vi "Keithley_pulse.vi"() -> ()   [LabVIEW 2023]
uses:
  <instrlib>/Keithley 24XX/Public/Data/Read (Multiple Points).vi
  <vilib>/Utility/file.llb/Write Delimited Spreadsheet (DBL).vi
  <instrlib>/Keithley 24XX/Keithley 24XX.lvlib
  <vilib>/Analysis/NI_AALBase.lvlib
panel:
  in  "valley milliseconds":u32=10
  in  "path1 (folder + filename)":string="C:\\Users\\Carter Fox\\Documents\\probe data\\haolin\\"
  in  "Clear Plot":bool
  out "V-R":cluster{dbl[], dbl[]}(graph)={[0.0, -0.5, -1.0, -1.5, -2.0, -2.5, -3.0, -3.5, -4.0, -3.5, -3.0, -2.5, -2.0, -1.5, -1.0, -0.5, 0.0, 0.5, 1.0, 1.5, 2.0, 2.5, 3.0, 3.5, 4.0, 3.5, 3.0, 2.5, 2.0, 1.5, 1.0, 0.5, 0.0, 0.0, -0.5, -1.0, -1.5, -2.0, -2.5, -3.0, -3.5, -4.0, -3.5, -3.0, -2.5, -2.0, -1.5, -1.0, -0.5, 0.0, 0.5, 1.0, 1.5, 2.0, 2.5, 3.0, 3.5, 4.0, 3.5, 3.0, 2.5, 2.0, 1.5, 1.0, 0.5, 0.0], [0.19700693041086198, 0.35372319519519807, 0.20753341913223267, 0.3582892343401909, 0.540878164768219, 0.43121315687894823, 0.1754639378748834, 0.002317465841770172, 0.0942357487976551, 0.08408013060688972, -0.1210348054766655, 0.06776629239320756, 0.04069728031754494, -0.04053474152460694, -0.23445252031087876, -0.3108171131461859, -25.74827651977539, -25.785472869873047, -25.82678337097168, -25.68000602722168, -25.46846694946289, -25.3049674987793, -25.380819702148436, -25.68810615539551, -25.51903533935547, -25.389516067504882, -25.12458267211914, -25.099736404418945, -25.550616455078124, -25.390170669555665, -25.549488830566407, -25.412010192871094, 0.08227393236011267, -0.25657982677221297, -0.08616339890286326, -0.01899189129471779, -0.26742409020662306, -0.07599621266126633, -0.11147867683321237, -0.09915755027905107, -0.13367668855935336, 0.060095877200365064, -0.09875441491603851, 0.18304548561573028, 0.24648103043437003, 0.05984655544161797, -0.01924160271883011, -0.14573073834180833, -0.221831959951669, -25.54925956726074, -25.60353775024414, -24.910662841796874, -25.843761825561522, -25.492467880249023, -26.035901641845705, -25.818101501464845, -25.60927963256836, -25.978542709350585, -25.790420913696288, -25.73311767578125, -26.193365859985352, -25.49853630065918, -25.56501159667969, -25.275862884521484, -25.529310989379884, -25.196596527099608]}
  in  "Sample Count":i32=5
  out "R error":dbl=0.15830408316018257 format="%0.2f"
  out "R":dbl=0.19700693041086198 format="%0.2f"
  in  "Source Mode  (0: Voltage)":u16(ring) items=["Voltage", "Current"]
  in  "Compliance  Level":dbl=1e-06
  in  "hill milliseconds":u32=10
  in  "Serial Configuration":T1={"Baud Rate"=9600, "Parity"=0, "Data Bits"=8, "Stop Bits"=10, "Flow Control"=0} {"Flow Control" items=["None", "XON/XOFF", "RTS/CTS", "XON/XOFF & RTS/CTS", "DTR/DSR", "XON/XOFF & DTR/DSR"]; "Stop Bits" items=["1.0"=10, "1.5"=15, "2.0"=20]; "Data Bits" items=["7"=7, "8"=8]; "Parity" items=["None", "Odd", "Even", "Mark", "Space"]; "Baud Rate" items=["300"=300, "600"=600, "1200"=1200, "2400"=2400, "4800"=4800, "9600"=9600, "19200"=19200]}
  in  "VISA resource name":refnum<visa-resource-name>="GPIB0::16::INSTR"
  in  "End Point 1 (V/A)":dbl=4.0
  in  "Region 2":bool
  in  "End Point 2 (V/A)":dbl=4.0
  in  "Step 2 (mV/mA)":dbl=500.0
  in  "Step 1 (mV/mA)":dbl=500.0
  in  "Starting Point (V/A)":dbl
  in  "Single/Double":i32=2 min=1 max=2 step=1
  out "Backward":bool
  out "Forward":bool=TRUE
  out "Region 1 steps":dbl=8.0
  out "Region 2  steps":dbl
  out "loop run":i32=2
  in  "loop #":i32=2
  in  "Save data or not":bool
  out "SD voltage":dbl format="%#_13g"
  # "Keithley Setting"
  # "Sweeping Setting"
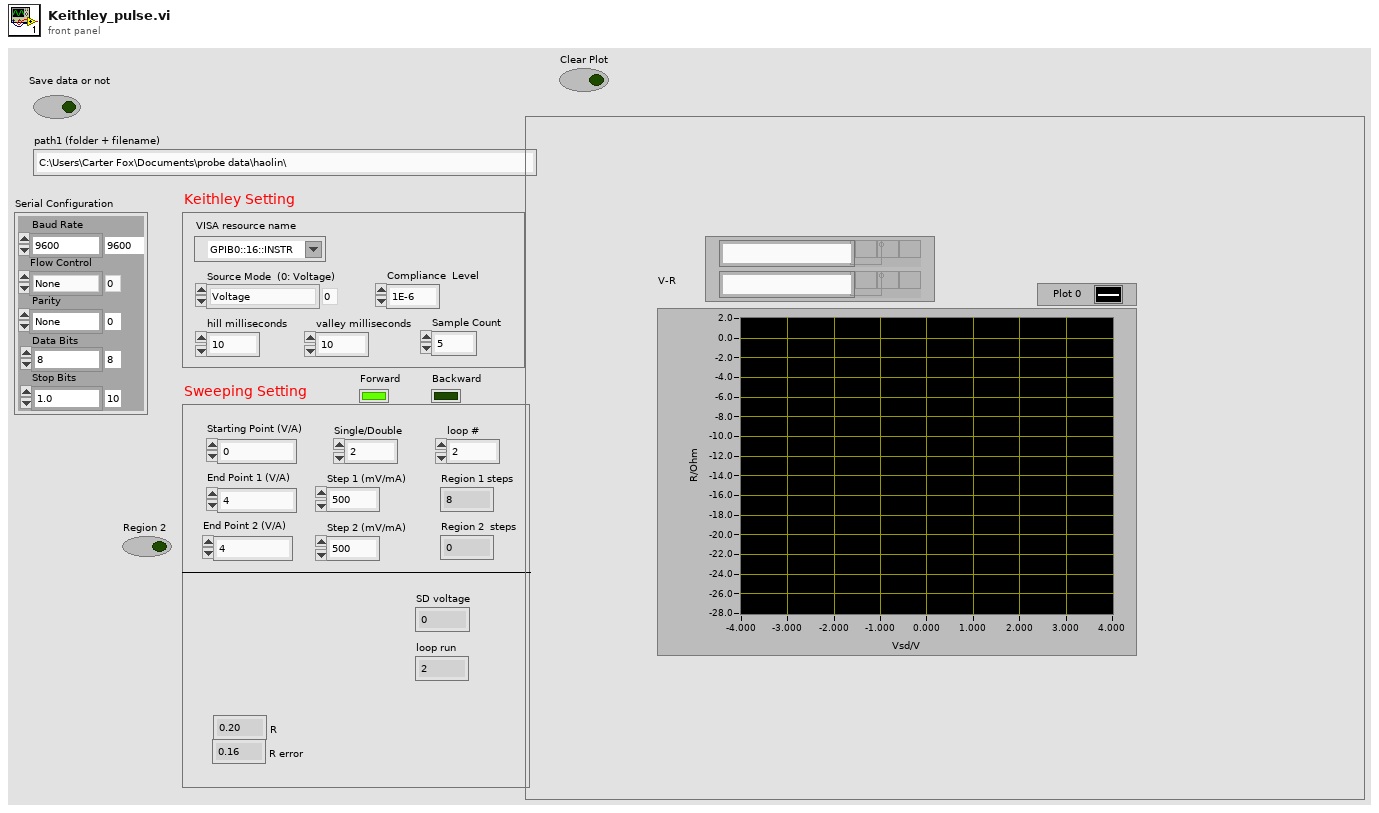
[diagram p1: front panel]
types:
  T1 = cluster{"Baud Rate":u32, "Parity":u16, "Data Bits":u16, "Stop Bits":u16, "Flow Control":u16}
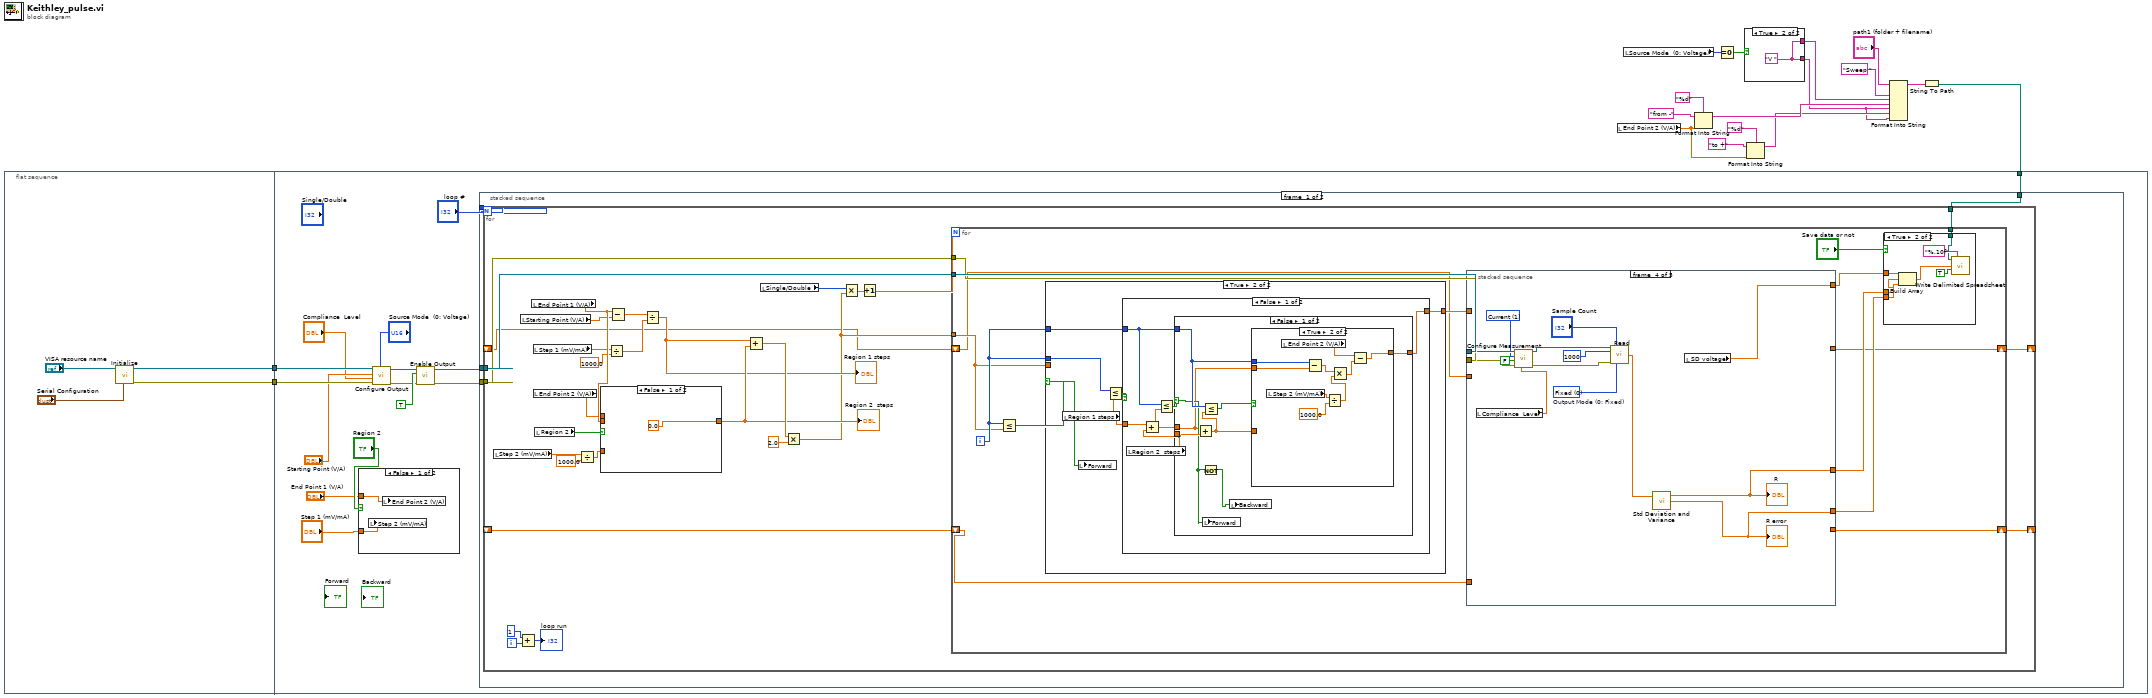
[diagram p0: block diagram]
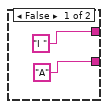
[diagram p2: hidden frame]
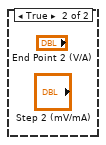
[diagram p3: hidden frame]
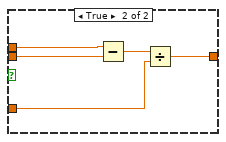
[diagram p4: hidden frame]
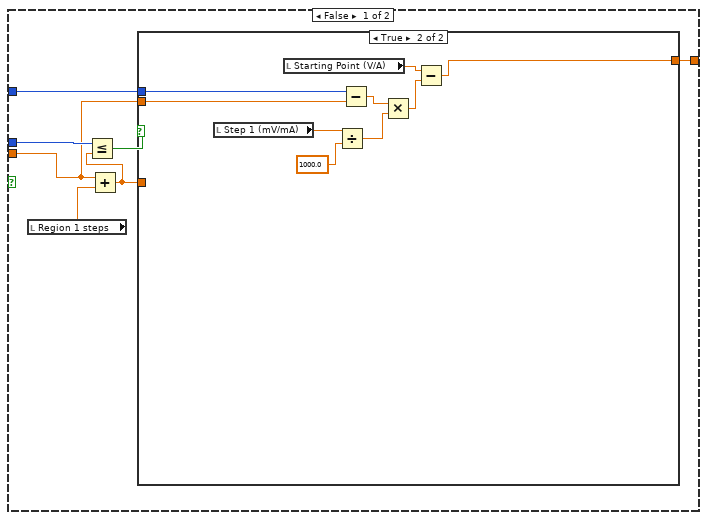
[diagram p5: hidden frame]
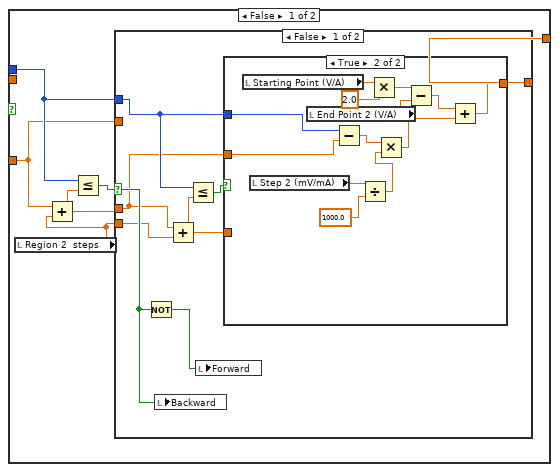
[diagram p6: hidden frame]
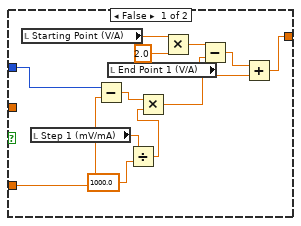
[diagram p7: hidden frame]
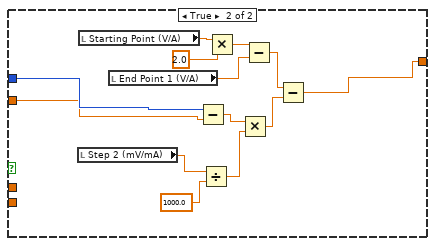
[diagram p8: hidden frame]
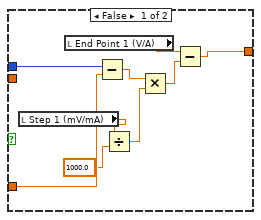
[diagram p9: hidden frame]
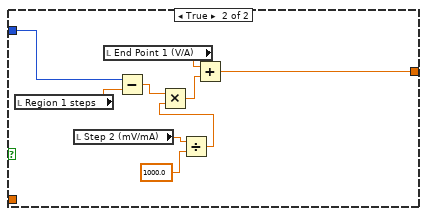
[diagram p10: hidden frame]
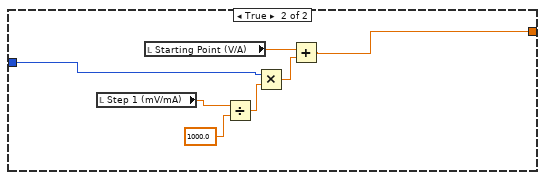
[diagram p11: hidden frame]
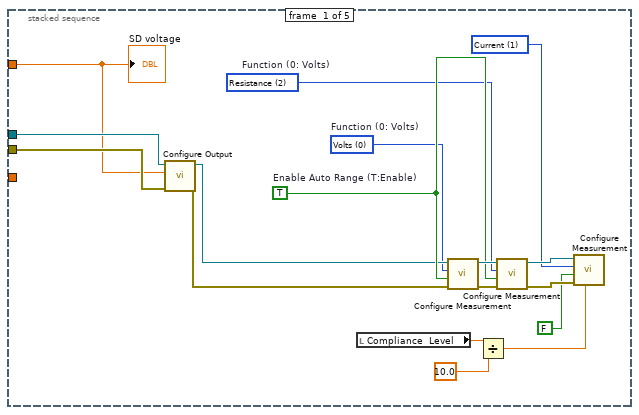
[diagram p13: hidden frame]
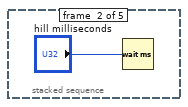
[diagram p14: hidden frame]
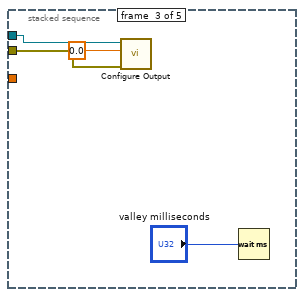
[diagram p15: hidden frame]
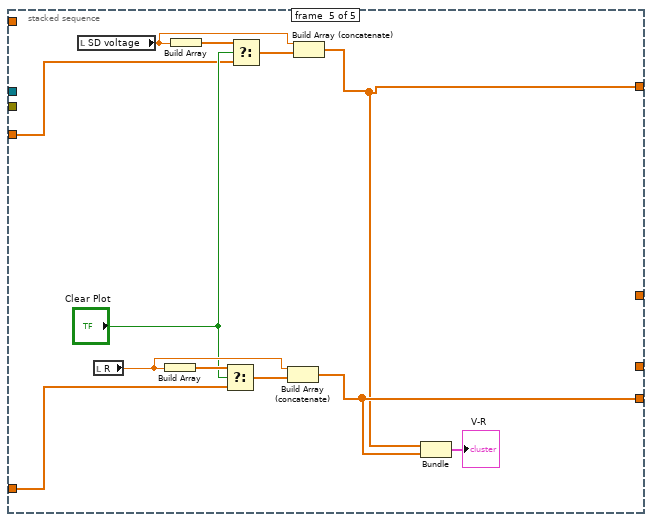
[diagram p16: hidden frame]
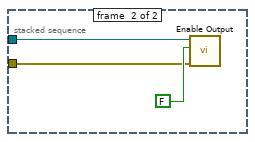
[diagram p17: hidden frame]
diagram:
  n1 = flat-sequence {
    tunnel: [w19] -> w17
    tunnel: [w18] -> w16
    tunnel: w17 -> [w29]
    tunnel: w16 -> [w28]
    tunnel: w13 -> [w22]
    frame #0 {
      n2 = call <instrlib>:"Initialize.vi"("Serial Configuration"="Serial Configuration", "VISA resource name"="VISA resource name") -> ("error out"=w18:errorcluster, "VISA resource name out"=w19:refnum<visa-resource-name>)  [unwired: 8 in]
    }
    frame #1 {
      n3 = case shown="False" "Region 2" {
        tunnel: "End Point 1 (V/A)" -> [w38 _]
        tunnel: "Step 1 (mV/mA)" -> [w37 _]
        frame False {
          n4 = local write "Step 2 (mV/mA)"(w37) -> ()
          n5 = local write "End Point 2 (V/A)"(w38) -> ()
        }
        frame True {
        }
      }
      n6 = call <instrlib>:"Configure Output.vi"("Source Mode  (0: Voltage)"="Source Mode  (0: Voltage)", "error in (no error)"=w28, "Compliance  Level (0.1)"="Compliance  Level", "Output Level (0)"="Starting Point (V/A)", "VISA resource name"=w29) -> ("error out"=w31:errorcluster, "VISA resource name out"=w30:refnum<visa-resource-name>)  [unwired: 5 in]
      n7 = call <instrlib>:"Enable Output.vi"("error in (no error)"=w31, "Enable Output (T: Enable)"=TRUE, "VISA resource name"=w30) -> ("error out"=w26:errorcluster, "VISA resource name out"=w27:refnum<visa-resource-name>)  [unwired: 7 in]
      n8 = stacked-sequence {
        tunnel: "loop #" -> [w42 _]
        tunnel: w27 -> [w41 w272]
        tunnel: w26 -> [w40 w271]
        tunnel: w22 -> [w39 _]
        frame #0 {
          n9 = for {
            N: w42 -> [_]
            tunnel: w41 -> [w71]
            tunnel: w40 -> [w54]
            shift-right: [w47] -> _
            shift-left: _ -> [w46]
            tunnel: w39 -> [w45]
            shift-right: [w44] -> _
            shift-left: _ -> [w43]
            i -> [w69]
            n10 = local read "Step 2 (mV/mA)"() -> (w50:dbl)
            n11 = Add(x=1, y=w69) -> (x+y=→"loop run":i32)
            n12 = local read "Starting Point (V/A)"() -> (w64:dbl)
            n13 = local read "End Point 1 (V/A)"() -> (w66:dbl)
            n14 = local read "Step 1 (mV/mA)"() -> (w51:dbl)
            n15 = local read "End Point 2 (V/A)"() -> (w65:dbl)
            n16 = local read "Region 2"() -> (w61:bool)
            n17 = Divide(x=w50, y=1000.0) -> (x/y=w48:dbl)
            n18 = case shown="False" w61 {
              tunnel: w66 -> [_ w76]
              tunnel: [0.0 w75] -> w63
              tunnel: w48 -> [_ w74]
              tunnel: w65 -> [_ w73]
              frame False {
              }
              frame True {
                n19 = Subtract(x=w73, y=w76) -> (x-y=w77:dbl)
                n20 = Divide(x=w77, y=w74) -> (x/y=w75:dbl)
              }
            }
            "Region 2  steps" <- w63
            n21 = Divide(x=w51, y=1000.0) -> (x/y=w53:dbl)
            n22 = Subtract(x=w66, y=w64) -> (x-y=w58:dbl)
            n23 = Divide(x=w58, y=w53) -> (x/y=w62:dbl)
            "Region 1 steps" <- w62
            n24 = Add(x=w62, y=w63) -> (x+y=w67:dbl)
            n25 = local read "Single/Double"() -> (w60:i32)
            n26 = Multiply(x=w67, y=2.0) -> (x*y=w55:dbl)
            n27 = Multiply(x=w60, y=w55) -> (x*y=w59:dbl)
            n28 = Increment(x=w59) -> (x+1=w56:dbl)
            n29 = for {
              N: w56 -> [_]
              tunnel: w71 -> [w92]
              tunnel: w55 -> [w88]
              tunnel: w54 -> [w86]
              shift-right: [w85] -> w47
              shift-left: w46 -> [w84]
              tunnel: w45 -> [w80]
              shift-right: [w79] -> w44
              shift-left: w43 -> [w78]
              i -> [w89]
              n30 = Less Or Equal?(x=w89, y=w88) -> (x <= y?=w90:bool)
              n31 = case shown="True" w90 {
                selector: w90 -> [_ w163]
                tunnel: w89 -> [w99 w167]
                tunnel: [w95 w166] -> w87
                tunnel: w89 -> [w98 w165]
                tunnel: w88 -> [w94 _]
                frame False {
                  n32 = local read "Region 1 steps"() -> (w96:dbl)
                  n33 = Add(x=w94, y=w96) -> (x+y=w93:dbl)
                  n34 = Less Or Equal?(x=w98, y=w93) -> (x <= y?=w97:bool)
                  n35 = case shown="True" w97 {
                    tunnel: w99 -> [w103 w161]
                    tunnel: [w104 w158] -> w95
                    tunnel: w94 -> [_ w157]
                    tunnel: w93 -> [w102 _]
                    frame False {
                      n36 = local read "Region 2  steps"() -> (w100:dbl)
                      n37 = Add(x=w102, y=w100) -> (x+y=w101:dbl)
                      n38 = Less Or Equal?(x=w103, y=w101) -> (x <= y?=w105:bool)
                      n39 = case shown="False" w105 {
                        selector: w105 -> [w112 _]
                        tunnel: [w113 w152] -> w104
                        tunnel: w103 -> [w108 w151]
                        tunnel: w102 -> [_ w150]
                        tunnel: w101 -> [w107 _]
                        tunnel: w100 -> [w109 _]
                        frame False {
                          n40 = Not(x=w112) -> (.not. x?=w111:bool)
                          n41 = local write "Backward"(w112) -> ()
                          n42 = Add(x=w107, y=w109) -> (x+y=w106:dbl)
                          n43 = Less Or Equal?(x=w108, y=w106) -> (x <= y?=w110:bool)
                          n44 = local write "Forward"(w111) -> ()
                          n45 = case shown="True" w110 {
                            tunnel: [w123 w138] -> w113
                            tunnel: w108 -> [w122 w137]
                            tunnel: w107 -> [_ w136]
                            tunnel: w106 -> [w121 _]
                            frame False {
                              n46 = local read "Starting Point (V/A)"() -> (w119:dbl)
                              n47 = local read "Step 1 (mV/mA)"() -> (w115:dbl)
                              n48 = Subtract(x=w122, y=w121) -> (x-y=w120:dbl)
                              n49 = local read "End Point 1 (V/A)"() -> (w117:dbl)
                              n50 = Divide(x=w115, y=1000.0) -> (x/y=w114:dbl)
                              n51 = Multiply(x=w120, y=w114) -> (x*y=w126:dbl)
                              n52 = Multiply(x=w119, y=2.0) -> (x*y=w125:dbl)
                              n53 = Subtract(x=w125, y=w117) -> (x-y=w124:dbl)
                              n54 = Add(x=w124, y=w126) -> (x+y=w123:dbl)
                            }
                            frame True {
                              n55 = local read "Starting Point (V/A)"() -> (w133:dbl)
                              n56 = local read "Step 2 (mV/mA)"() -> (w128:dbl)
                              n57 = local read "End Point 2 (V/A)"() -> (w130:dbl)
                              n58 = Subtract(x=w137, y=w136) -> (x-y=w131:dbl)
                              n59 = Divide(x=w128, y=1000.0) -> (x/y=w127:dbl)
                              n60 = Multiply(x=w133, y=2.0) -> (x*y=w135:dbl)
                              n61 = Multiply(x=w131, y=w127) -> (x*y=w139:dbl)
                              n62 = Subtract(x=w135, y=w130) -> (x-y=w134:dbl)
                              n63 = Add(x=w134, y=w139) -> (x+y=w138:dbl)
                            }
                          }
                        }
                        frame True {
                          n64 = local read "Step 2 (mV/mA)"() -> (w141:dbl)
                          n65 = local read "Starting Point (V/A)"() -> (w146:dbl)
                          n66 = local read "End Point 1 (V/A)"() -> (w144:dbl)
                          n67 = Subtract(x=w151, y=w150) -> (x-y=w148:dbl)
                          n68 = Divide(x=w141, y=1000.0) -> (x/y=w140:dbl)
                          n69 = Multiply(x=w146, y=2.0) -> (x*y=w147:dbl)
                          n70 = Multiply(x=w148, y=w140) -> (x*y=w149:dbl)
                          n71 = Subtract(x=w147, y=w144) -> (x-y=w143:dbl)
                          n72 = Subtract(x=w143, y=w149) -> (x-y=w152:dbl)
                        }
                      }
                    }
                    frame True {
                      n73 = local read "Step 1 (mV/mA)"() -> (w154:dbl)
                      n74 = local read "Starting Point (V/A)"() -> (w159:dbl)
                      n75 = Divide(x=w154, y=1000.0) -> (x/y=w153:dbl)
                      n76 = Subtract(x=w161, y=w157) -> (x-y=w156:dbl)
                      n77 = Multiply(x=w156, y=w153) -> (x*y=w160:dbl)
                      n78 = Subtract(x=w159, y=w160) -> (x-y=w158:dbl)
                    }
                  }
                }
                frame True {
                  n79 = local read "Region 1 steps"() -> (w162:dbl)
                  n80 = local write "Forward"(w163) -> ()
                  n81 = Less Or Equal?(x=w165, y=w162) -> (x <= y?=w164:bool)
                  n82 = case shown="False" w164 {
                    tunnel: w167 -> [w171 w213]
                    tunnel: [w170 w214] -> w166
                    tunnel: w162 -> [w172 _]
                    frame False {
                      n83 = local read "Region 2  steps"() -> (w168:dbl)
                      n84 = Add(x=w172, y=w168) -> (x+y=w169:dbl)
                      n85 = Less Or Equal?(x=w171, y=w169) -> (x <= y?=w173:bool)
                      n86 = case shown="False" w173 {
                        selector: w173 -> [w177 _]
                        tunnel: w171 -> [w180 w206]
                        tunnel: [w181 w203] -> w170
                        tunnel: w169 -> [w175 _]
                        tunnel: w168 -> [w179 _]
                        frame False {
                          n87 = Add(x=w175, y=w179) -> (x+y=w174:dbl)
                          n88 = Not(x=w177) -> (.not. x?=w176:bool)
                          n89 = Less Or Equal?(x=w180, y=w174) -> (x <= y?=w178:bool)
                          n90 = local write "Forward"(w177) -> ()
                          n91 = local write "Backward"(w176) -> ()
                          n92 = case shown="True" w178 {
                            tunnel: w180 -> [w187 w196]
                            tunnel: [w185 w195] -> w181
                            tunnel: w175 -> [_ w194]
                            tunnel: w174 -> [w186 _]
                            frame False {
                              n93 = local read "Step 1 (mV/mA)"() -> (w183:dbl)
                              n94 = local read "End Point 1 (V/A)"() -> (w188:dbl)
                              n95 = Subtract(x=w187, y=w186) -> (x-y=w190:dbl)
                              n96 = Divide(x=w183, y=1000.0) -> (x/y=w182:dbl)
                              n97 = Multiply(x=w190, y=w182) -> (x*y=w189:dbl)
                              n98 = Subtract(x=w188, y=w189) -> (x-y=w185:dbl)
                            }
                            frame True {
                              n99 = local read "Step 2 (mV/mA)"() -> (w192:dbl)
                              n100 = local read "End Point 2 (V/A)"() -> (w197:dbl)
                              n101 = Subtract(x=w196, y=w194) -> (x-y=w199:dbl)
                              n102 = Divide(x=w192, y=1000.0) -> (x/y=w191:dbl)
                              n103 = Multiply(x=w199, y=w191) -> (x*y=w198:dbl)
                              n104 = Subtract(x=w197, y=w198) -> (x-y=w195:dbl)
                            }
                          }
                        }
                        frame True {
                          n105 = local read "Region 1 steps"() -> (w205:dbl)
                          n106 = local read "Step 2 (mV/mA)"() -> (w202:dbl)
                          n107 = local read "End Point 1 (V/A)"() -> (w207:dbl)
                          n108 = Subtract(x=w206, y=w205) -> (x-y=w204:dbl)
                          n109 = Divide(x=w202, y=1000.0) -> (x/y=w200:dbl)
                          n110 = Multiply(x=w204, y=w200) -> (x*y=w208:dbl)
                          n111 = Add(x=w207, y=w208) -> (x+y=w203:dbl)
                        }
                      }
                    }
                    frame True {
                      n112 = local read "Step 1 (mV/mA)"() -> (w210:dbl)
                      n113 = local read "Starting Point (V/A)"() -> (w212:dbl)
                      n114 = Divide(x=w210, y=1000.0) -> (x/y=w209:dbl)
                      n115 = Multiply(x=w213, y=w209) -> (x*y=w215:dbl)
                      n116 = Add(x=w212, y=w215) -> (x+y=w214:dbl)
                    }
                  }
                }
              }
              n117 = stacked-sequence {
                tunnel: w92 -> [w238 _ w244 w252 _]
                tunnel: w86 -> [w239 _ w243 w251 _]
                tunnel: w87 -> [w237 _ _ _ _]
                tunnel: w78 -> [_ _ _ _ w260]
                tunnel: [_ _ _ _ w262] -> w85
                tunnel: w84 -> [_ _ _ _ w261]
                tunnel: [_ _ _ w245 _] -> w83
                tunnel: [_ _ _ w254 _] -> w82
                tunnel: [_ _ _ w253 _] -> w81
                tunnel: [_ _ _ _ w259] -> w79
                frame #0 {
                  w231 = u16 1 items=["Volts", "Current", "Resistance"] ("Function (0: Volts)")
                  w232 = TRUE  # Enable Auto Range (T:Enable)
                  w230 = u16 2 items=["Volts", "Current", "Resistance"]  # Function (0: Volts)
                  w227 = u16 0 items=["Volts", "Current", "Resistance"]  # Function (0: Volts)
                  n118 = call <instrlib>:"Configure Output.vi"("error in (no error)"=w239, "Output Level (0)"=w237, "VISA resource name"=w238) -> ("error out"=w228:errorcluster, "VISA resource name out"=w229:refnum<visa-resource-name>)  [unwired: 7 in]
                  n119 = local read "Compliance  Level"() -> (w225:dbl)
                  n120 = call <instrlib>:"Configure Measurement.vi"("error in (no error)"=w228, "Enable Auto Range (T:Enable)"=w232, "Function (0: Volts)"=w227, "VISA resource name"=w229) -> ("error out"=w233:errorcluster, "VISA resource name out"=w234:refnum<visa-resource-name>)  [unwired: 6 in]
                  n121 = Divide(x=w225, y=10.0) -> (x/y=w223:dbl)
                  n122 = call <instrlib>:"Configure Measurement.vi"("error in (no error)"=w233, "Enable Auto Range (T:Enable)"=w232, "Function (0: Volts)"=w230, "VISA resource name"=w234) -> ("error out"=w236:errorcluster, "VISA resource name out"=w235:refnum<visa-resource-name>)  [unwired: 6 in]
                  n123 = call <instrlib>:"Configure Measurement.vi"("Manual Range (1.0)"=w223, "error in (no error)"=w236, "Enable Auto Range (T:Enable)"=FALSE, "Function (0: Volts)"=w231, "VISA resource name"=w235) -> ()  [unwired: 5 in, 2 out]
                  "SD voltage" <- w237
                }
                frame #1 {
                  n124 = Wait (ms)(milliseconds to wait="hill milliseconds") -> ()  [unwired: 1 out]
                }
                frame #2 {
                  n125 = call <instrlib>:"Configure Output.vi"("error in (no error)"=w243, "Output Level (0)"=0.0, "VISA resource name"=w244) -> ()  [unwired: 7 in, 2 out]
                  n126 = Wait (ms)(milliseconds to wait="valley milliseconds") -> ()  [unwired: 1 out]
                }
                frame #3 {
                  w248 = u16 1 items=["Volts", "Current", "Resistance"] ("Function (0: Volts)")
                  w257 = u16 0 items=["Fixed", "Sweep", "List"]  # Output Mode (0: Fixed)
                  n127 = local read "Compliance  Level"() -> (w246:dbl)
                  n128 = call <instrlib>:"Configure Measurement.vi"("Manual Range (1.0)"=w246, "error in (no error)"=w251, "Enable Auto Range (T:Enable)"=FALSE, "Function (0: Volts)"=w248, "VISA resource name"=w252) -> ("error out"=w250:errorcluster, "VISA resource name out"=w249:refnum<visa-resource-name>)  [unwired: 5 in]
                  n129 = call-poly <instrlib>:"Read.vi"("VISA resource name"=w249, "Sample Count (1)"="Sample Count", "Timeout (10000 ms)"=1000, "error in (no error)"=w250, "Output Mode (0: Fixed)"=w257) -> ("Resistance"=w256:sgl[])  [unwired: 4 in, 6 out]
                  n130 = call <vilib>:"Std Deviation and Variance.vi"("X"=w256) -> ("mean"=w254:dbl, "standard deviation"=w253:dbl)  [unwired: 1 in, 1 out]
                  "R" <- w254
                  "R error" <- w253
                  n131 = local read "SD voltage"() -> (w245:dbl)
                }
                frame #4 {
                  n132 = local read "SD voltage"() -> (w269:dbl)
                  n133 = local read "R"() -> (w264:dbl)
                  n134 = Build Array(w264) -> (w266:dbl[])
                  n135 = Build Array(w269) -> (w270:dbl[])
                  n136 = Select(t=w266, s="Clear Plot", f=w261) -> (s? t:f=w265:dbl[])
                  n137 = Select(t=w270, s="Clear Plot", f=w260) -> (s? t:f=w268:dbl[])
                  n138 = Build Array (concatenate)(w264, w265) -> (w262:dbl[])
                  n139 = Build Array (concatenate)(w269, w268) -> (w259:dbl[])
                  n140 = Bundle(w259, w262) -> (→"V-R":cluster{dbl[], dbl[]})  [unwired: 1 in]
                }
              }
              n141 = case shown="True" "Save data or not" {
                tunnel: w83 -> [_ w219]
                tunnel: w82 -> [_ w216]
                tunnel: w81 -> [_ w217]
                tunnel: w80 -> [_ w218]
                frame False {
                }
                frame True {
                  n142 = Build Array(w219, w216, w217) -> (w222:dbl[])
                  n143 = call-poly <vilib>:"Write Delimited Spreadsheet.vi"("file path (dialog if empty)"=w218, "format (%.3f)"="%.10f", "1D data"=w222, "append to file? (new file:F)"=TRUE) -> ()  [unwired: 10 in, 2 out]
                }
              }
            }
          }
        }
        frame #1 {
          n144 = call <instrlib>:"Enable Output.vi"("error in (no error)"=w271, "Enable Output (T: Enable)"=FALSE, "VISA resource name"=w272) -> ()  [unwired: 7 in, 2 out]
        }
      }
    }
  }
  n145 = local read "End Point 2 (V/A)"() -> (w3:dbl)
  n146 = local read "Source Mode  (0: Voltage)"() -> (w12:u16)
  n147 = Format Into String(format string="%d", initial string="from -", w3) -> (resulting string=w6:string)  [unwired: 1 in, 1 out]
  n148 = Equal To 0?(x=w12) -> (x = 0?=w11:bool)
  n149 = case shown="True" w11 {
    tunnel: ["I " ("input 1") w276] -> w9
    tunnel: ["A" ("input 1") w276] -> w1
    frame False {
    }
    frame True {
      w276 = "V " ("input 1")
    }
  }
  n150 = Format Into String(format string="%d", initial string="to +", w3) -> (resulting string=w2:string)  [unwired: 1 in, 1 out]
  n151 = Format Into String(initial string="path1 (folder + filename)", "Sweep " ("input 1"), w9, w6, w1, w2, w1) -> (resulting string=w14:string)  [unwired: 2 in, 1 out]
  n152 = String To Path(string=w14) -> (path=w13:path)
